vi "Configure Trigger.vi"(8 "error in (no error)":errorcluster, 10 "Trigger Source (0: Internal)":u16(ring) items=["Internal", "External", "Software (bus)"], 11 "VISA resource name":refnum<visa-resource-name>) -> (0 "error out":errorcluster, 3 "VISA resource name out":refnum<visa-resource-name>)   [LabVIEW 2013, in "Template - Function Generator.lvlib"]
doc: "Configures the trigger source for triggering sweeps.\n\n<B>Note:</B> Use this VI only with other low-level VIs. The high-level VIs automatically incorporate this functionality. This VI does not check the instrument status. If you want to check the instrument status, call the Error Query VI at the conclusion of your sweep operation."
uses:
  <instrlib>/_Template - Function Generator/Template - Function Generator.lvlib
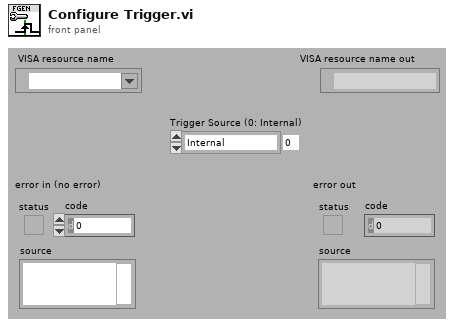
[diagram p1: front panel]
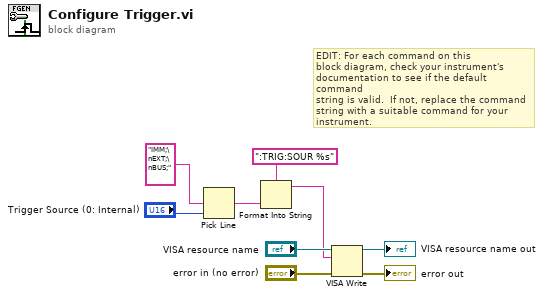
[diagram p0: block diagram]
diagram:
  # "EDIT: For each command on this\nblock diagram, check your instrument's\ndocumentation to see if the default command\nstring is valid.  If not, replace the command\nstring with a suitable command for your\ninstrument."
  n1 = Pick Line(multi-line string="IMM;\nEXT;\nBUS;", line index="Trigger Source (0: Internal)") -> (output string=w5:string)  [unwired: 1 in]
  n2 = Format Into String(format string=":TRIG:SOUR %s", w5) -> (resulting string=w3:string)  [unwired: 2 in, 1 out]
  n3 = VISA Write(VISA resource name="VISA resource name", write buffer=w3, error in (no error)="error in (no error)") -> (VISA resource name out=→"VISA resource name out":refnum<visa-resource-name>, error out=→"error out":errorcluster)  [unwired: 1 out]
